vi "PipBoy_ChangeActiveLabVIEW.vi"(8 "error in (no error)":errorcluster, 10 "LvVersion":string, 11 "PipBoyDataIn":T1) -> (0 "error out":errorcluster, 3 "PipBoyDataOut":T1)   [LabVIEW 2014]
uses:
  ctls/PipBoy_PipBoyData.ctl
  ctls/PipBoy_ProcComm.ctl
  System.Windows.Forms
  ctls/PipBoy_PipBoyCommand.ctl
  ctls/PipBoy_Message.ctl
  modules/support/Message Queue/All Message Queues.ctl
  modules/support/Message Queue/Message Cluster.ctl
  ctls/PipBoy_FileConf.ctl
  ctls/PipBoy_PicComm.ctl
  ctls/PipBoy_GeneralParams.ctl
  ctls/PipBoy_Pages.ctl
  modules/support/Message Queue/Message Queue.lvlib
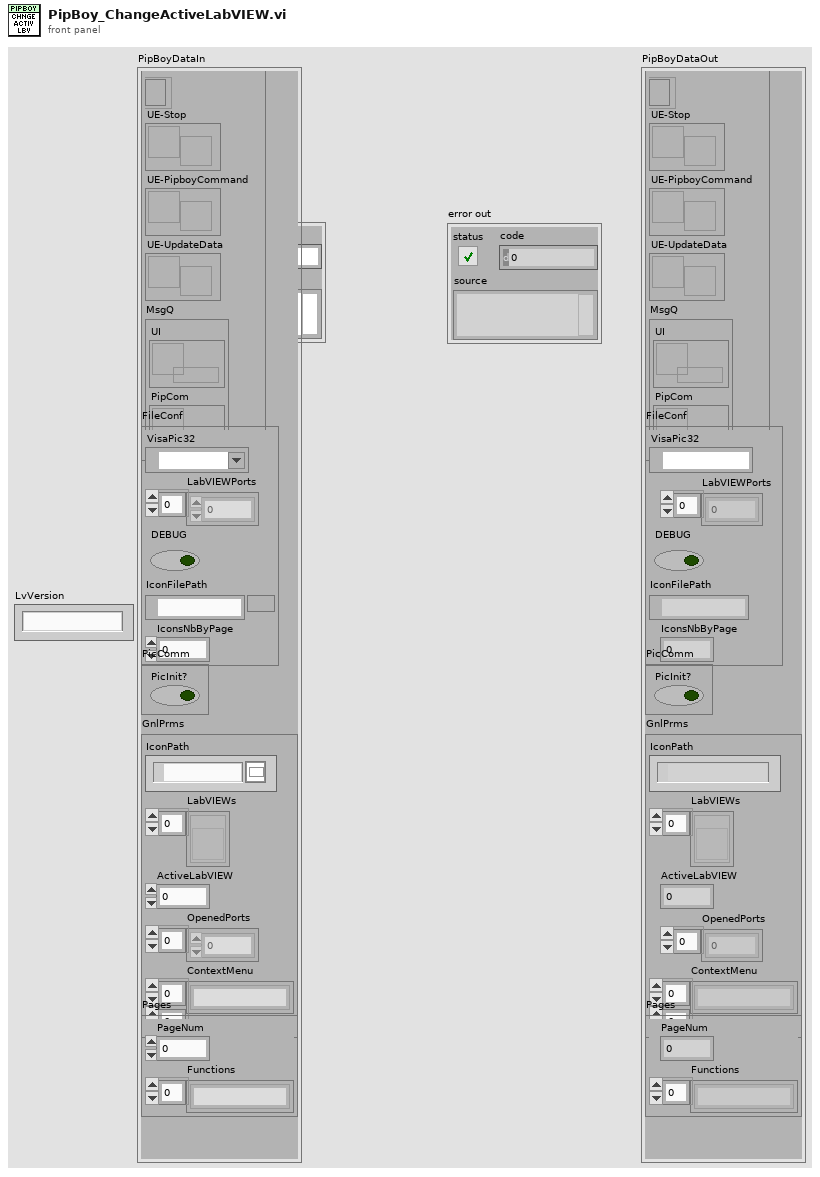
[diagram p1: front panel]
types:
  T1 = typedef "PipBoy_PipBoyData.ctl" = cluster{"ProcComm":T2, "FileConf":T4, "PicComm":T5, "GnlPrms":T6, "Pages":T7}
  T2 = typedef "PipBoy_ProcComm.ctl" = cluster{"NotifyIconRef":refnum<k24>, "UE-Stop":refnum<user-event>, "UE-PipboyCommand":refnum<user-event>, "UE-UpdateData":refnum<user-event>, "MsgQ":T3}
  T3 = typedef "Message Queue.lvlib/All Message Queues.ctl" = cluster{"UI":refnum<queue>, "PipCom":refnum<queue>}
  T4 = typedef "PipBoy_FileConf.ctl" = cluster{"VisaPic32":refnum<visa-resource-name>, "LabVIEWPorts":u16[], "DEBUG":bool, "IconFilePath":path, "IconsNbByPage":i32}
  T5 = typedef "PipBoy_PicComm.ctl" = cluster{"PicInit?":bool}
  T6 = typedef "PipBoy_GeneralParams.ctl" = cluster{"IconPath":path, "LabVIEWs":refnum<vi>[], "ActiveLabVIEW":i32, "OpenedPorts":u16[], "ContextMenu":string[][]}
  T7 = typedef "PipBoy_Pages.ctl" = cluster{"PageNum":i32, "Functions":string[]}
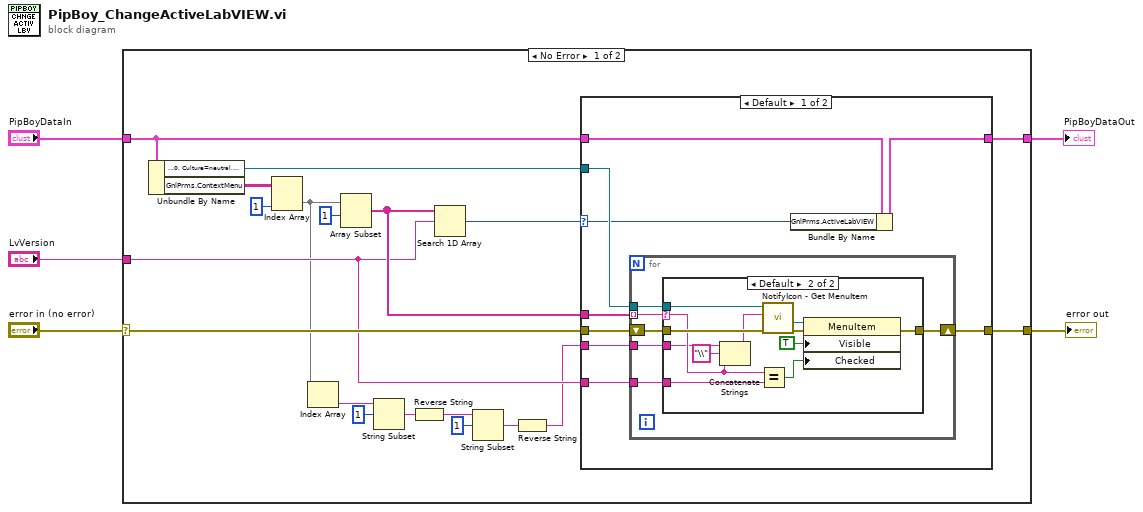
[diagram p0: block diagram]
diagram:
  n1 = case shown="No Error" "error in (no error)" {
    selector: "error in (no error)" -> [w19 w56]
    tunnel: [w18 w56] -> w4
    tunnel: "PipBoyDataIn" -> [w20 w55]
    tunnel: [w21 w55] -> w2
    tunnel: "LvVersion" -> [w14 _]
    frame No Error {
      n2 = Unbundle By Name(w20) -> ("ProcComm.NotifyIconRef"=w17:refnum<k24>, "GnlPrms.ContextMenu"=w24:string[][])
      n3 = Index Array(array=w24, index (col)=1 ("disabled index (col)")) -> (element=w7:string[])  [unwired: 1 in]
      n4 = Index Array(array=w7) -> (element=w8:string)  [unwired: 1 in]
      n5 = Array Subset(array=w7, index=1) -> (w15:string[])  [unwired: 1 in]
      n6 = String Subset(string=w8, offset (0)=1) -> (substring=w12:string)  [unwired: 1 in]
      n7 = Reverse String(1:w12) -> (0:w11:string)
      n8 = Search 1D Array(1D array=w15, element=w14) -> (index of element=w22:i32)  [unwired: 1 in]
      n9 = String Subset(string=w11, offset (0)=1) -> (substring=w9:string)  [unwired: 1 in]
      n10 = Reverse String(1:w9) -> (0:w6:string)
      n11 = case shown="Default" w22 {
        selector: w22 -> [w28 _]
        tunnel: w20 -> [w33 w54]
        tunnel: [w32 w54] -> w21
        tunnel: w19 -> [w31 w53]
        tunnel: [w30 w53] -> w18
        tunnel: w17 -> [w29 _]
        tunnel: w15 -> [w27 _]
        tunnel: w14 -> [w26 _]
        tunnel: w6 -> [w25 _]
        frame Default {
          n12 = for {
            tunnel: w29 -> [w37]
            shift-right: [w38] -> w30
            shift-left: w31 -> [w39]
            tunnel: w27 -> [w35] mode=indexing
            tunnel: w26 -> [w36]
            tunnel: w25 -> [w34]
            n13 = case shown="Default" w35 {
              selector: w35 -> [_ w42]
              tunnel: w39 -> [w40 w49]
              tunnel: [w40 w48] -> w38
              tunnel: w37 -> [_ w47]
              tunnel: w36 -> [_ w45]
              tunnel: w34 -> [_ w41]
              frame "\u0000" {
              }
              frame Default {
                n14 = Concatenate Strings(w41, "\\" ("element"), w42) -> (w43:string)
                n15 = Equal?(x=w42, y=w45) -> (x = y?=w46:bool)
                n16 = call <userlib>:"NotifyIcon - Get MenuItem.vi"("error in"=w49, "Context MenuItem"=w43, "NotifyIcon reference in"=w47) -> ("error out"=w52:errorcluster, "MenuItem reference"=w51:refnum<k24>)  [unwired: 6 in, 1 out]
                n17 = property class="MenuItem"(reference=w51, error in=w52, "Visible"=TRUE, "Checked"=w46) -> (error out=w48:errorcluster)  [unwired: 1 out]
              }
            }
          }
          n18 = Bundle By Name(cluster=w33, "GnlPrms.ActiveLabVIEW"=w28) -> (w32:T1)
        }
        frame -1 {
        }
      }
    }
    frame Error {
    }
  }
  "error out" <- w4
  "PipBoyDataOut" <- w2
